vi "get_voltage_set_low_limit.vi"(8 "error in":errorcluster, 11 "VISA resource name":refnum<visa-resource-name>="COM1") -> (0 "error out":errorcluster, 3 "Response":string)   [LabVIEW 2020]
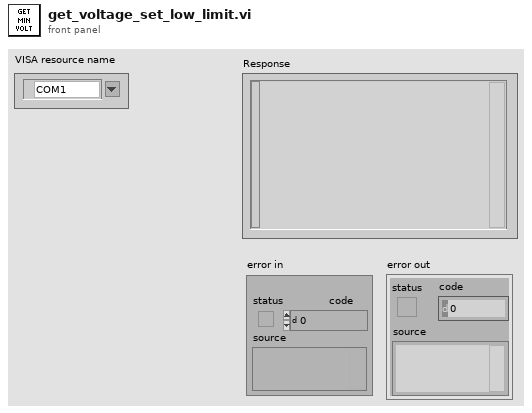
[diagram p1: front panel]
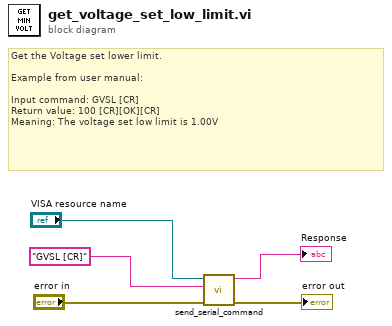
[diagram p0: block diagram]
diagram:
  # "Get the Voltage set lower limit.\n\nExample from user manual:\n\nInput command: GVSL [CR]\nReturn value: 100 [CR][OK][CR]\nMeaning: The voltage set low limit is 1.00V"
  n1 = call "send_serial_command.vi"("error in (no error)"="error in", "Command"="GVSL [CR]", "VISA resource name"="VISA resource name") -> ("error out"=→"error out":errorcluster, "Response"=→"Response":string)  [unwired: 7 in]
